vi "camera mjpeg.vi"(11 "CameraDevRef":T1) -> ()   [LabVIEW 2013]
uses:
  <vilib>/Rock Robotics/WPI/Camera/WPI_CameraDevRef.ctl
  <vilib>/Rock Robotics/WPI/Camera/WPI_CameraSettings Operations.ctl
  typedefs/fg_typedef.ctl
  typedefs/Vision/vision enable.ctl
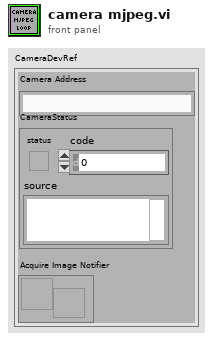
[diagram p1: front panel]
types:
  T1 = typedef "WPI_CameraDevRef.ctl" = cluster{"Camera Address":string, "CameraStatus":errorcluster, "Acquire Image Notifier":refnum<notifier>}
  T2 = typedef "WPI_CameraSettings Operations.ctl" = enum16{"Udate FPS", "Update Compression", "Update Size", "Update White Balance", "Update Brightness", "Update Sharpness", "Update Exposure", "Update Color Level", "Update Exp Priority", "Update Color Enable", "Update JPG", "Update MJPG", "Read and Clear", "Read", "Init"}
  T3 = typedef "vision enable.ctl" = enum16{"Enable", "Disable", "Stop"}
  T4 = typedef "fg_typedef.ctl" = enum16{"Get", "Set"}
  T5 = typedef "WPI_CameraSettings Control.ctl" = cluster{"FPS":i32, "Compression":i32, "Size":i32, "White Balance":i32, "Brightness":i32, "Sharpness":i32, "Exposure":i32, "Color Level":i32, "Exposure Priority":i32, "Color Enable":i32, "JPG Loop":i32, "MJPG Loop":i32}
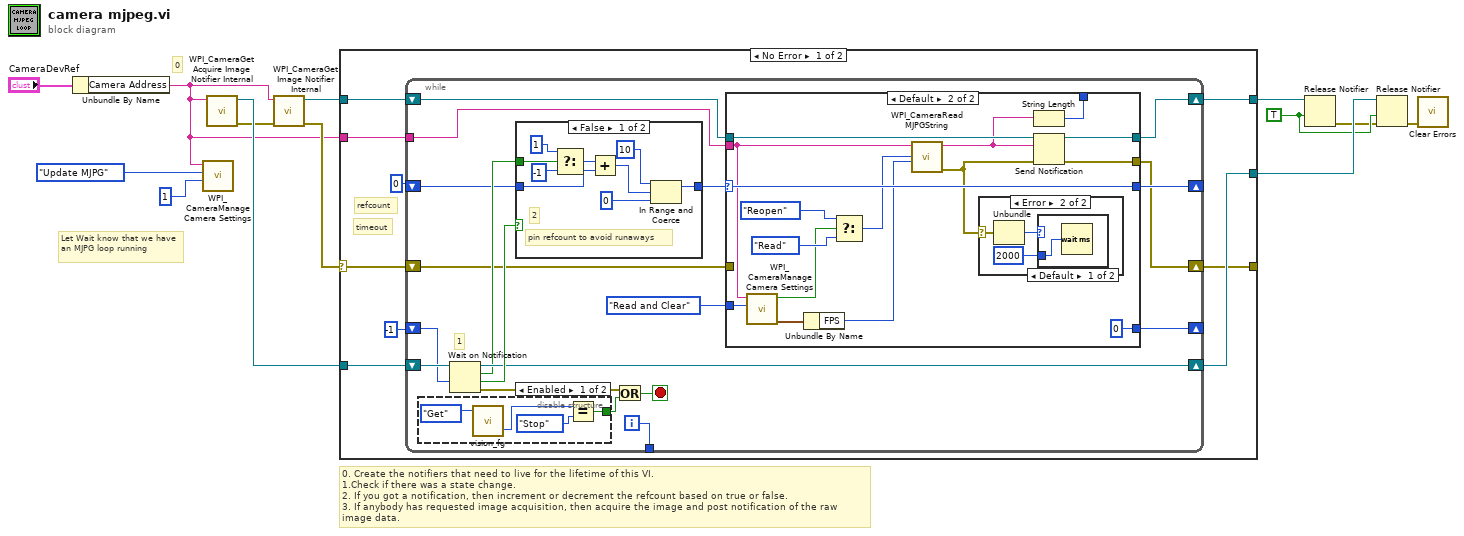
[diagram p0: block diagram]
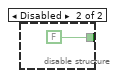
[diagram p2: hidden frame]
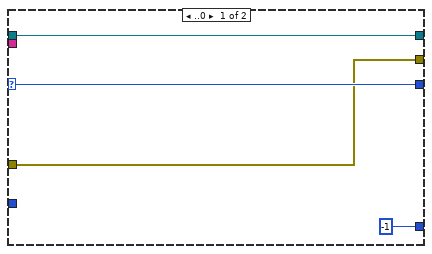
[diagram p3: hidden frame]
diagram:
  w10 = TRUE ("force destroy? (F)")
  # "Let Wait know that we have\nan MJPG loop running"
  # "0"
  # "0. Create the notifiers that need to live for the lifetime of this VI. \n1.Check if there was a state change.\n2. If you got a notification, then increment or decrement the refcount based on true or false.\n3. If anybody has requested image acquisition, then acquire the image and post notification of the raw image data."
  n1 = Unbundle By Name("CameraDevRef") -> ("Camera Address"=w1:string)
  n2 = call <vilib>:"WPI_CameraManage Camera Settings.vi"("Value"=1, "Operation"=WPI_CameraSettings_Operations."Update MJPG", "Camera IP"=w1) -> ()  [unwired: 7 in, 2 out]
  n3 = call <vilib>:"WPI_CameraGet Acquire Image Notifier Internal.vi"("Camera Address"=w1) -> ("error out"=w5:errorcluster, "Acquire Image Notifier"=w6:refnum<notifier>)  [unwired: 1 in, 8 out]
  n4 = call <vilib>:"WPI_CameraGet Image Notifier Internal.vi"("error in (no error)"=w5, "Camera Address"=w1) -> ("error out"=w8:errorcluster, "Image Notifier"=w11:refnum<notifier>)  [unwired: 8 out]
  n5 = case shown="No Error" w8 {
    selector: w8 -> [w15 w83]
    tunnel: w1 -> [w22 _]
    tunnel: w6 -> [w21 w81]
    tunnel: w11 -> [w19 w82]
    tunnel: [w17 w82] -> w13
    tunnel: [w16 w81] -> w12
    tunnel: [w14 w83] -> _
    frame No Error {
      # "timeout"
      # "refcount"
      n6 = while {
        shift-right: [w39] -> w16
        shift-left: w21 -> [w41]
        tunnel: w22 -> [w36]
        shift-right: [w29] -> _
        shift-left: 0 -> [w37]
        shift-right: [w34] -> w17
        shift-left: w19 -> [w35]
        shift-right: [w32] -> _
        shift-left: -1 -> [w33]
        shift-right: [w28] -> w14
        shift-left: w15 -> [w31]
        tunnel: [w26] -> _
        i -> [w26]
        stop <- w25 stop-if-true
        # "1"
        n7 = disable-structure shown="Enabled" {
          disable-tunnel: [w42 FALSE] -> w23
          frame Enabled {
            n8 = call "vision_fg.vi"("Menu"=fg_typedef."Get") -> ("State Out"=w44:T3)  [unwired: 2 in, 1 out]
            n9 = Equal?(x=w44, y=vision_enable."Stop") -> (x = y?=w42:bool)
          }
          frame Disabled {
          }
        }
        n10 = Wait on Notification(notifier=w41, timeout in ms (-1)=w33) -> (notifier out=w39:refnum<notifier>, notification=w38:bool, timed out?=w40:bool, error out=w24:errorcluster)  [unwired: 1 in, 1 out]
        n11 = case shown="False" w40 {
          tunnel: w38 -> [w79 _]
          tunnel: w37 -> [w75 w80]
          tunnel: [w71 w80] -> w30
          frame False {
            # "pin refcount to avoid runaways"
            # "2"
            n12 = Select(t=1, s=w79, f=-1) -> (s? t:f=w76:i32)
            n13 = Add(x=w76, y=w75) -> (x+y=w72:i32)
            n14 = In Range and Coerce(upper limit=10, x=w72, lower limit=0) -> (coerced(x)=w71:i32)  [unwired: 1 out]
          }
          frame True {
          }
        }
        n15 = Or(x=w24, y=w23) -> (x .or. y?=w25:bool)
        n16 = case shown="Default" w30 {
          selector: w30 -> [w49 w63]
          tunnel: w36 -> [_ w51]
          tunnel: w35 -> [w50 w66]
          tunnel: [w50 w65] -> w34
          tunnel: [-1 0] -> w32
          tunnel: w31 -> [w47 _]
          tunnel: [w49 w63] -> w29
          tunnel: [w47 w62] -> w28
          tunnel: [_ w56] -> _
          tunnel: WPI_CameraSettings_Operations."Read and Clear" ("Operation") -> [_ w52]
          frame ..0 {
          }
          frame Default {
            n17 = call <vilib>:"WPI_CameraManage Camera Settings.vi"("Operation"=w52, "Camera IP"=w51) -> ("Values"=w54:T5, "Changed"=w55:bool)  [unwired: 8 in]
            n18 = Unbundle By Name(w54) -> ("FPS"=w53:i32)
            n19 = Select(t=enum16{"Read", "Reopen", "Close"}."Reopen" ("Operation"), s=w55, f=enum16{"Read", "Reopen", "Close"}."Read" ("Operation")) -> (s? t:f=w58:enum16{"Read", "Reopen", "Close"})
            n20 = call <vilib>:"WPI_CameraRead MJPGString.vi"("fps"=w53, "Operation"=w58, "address"=w51) -> ("error out"=w61:errorcluster, "Raw Image Data"=w57:string)  [unwired: 7 in]
            n21 = case shown="Error" w61 {
              selector: w61 -> [_ w69]
              frame No Error {
              }
              frame Error {
                n22 = Unbundle(w69) -> ("code"=w68:i32)  [unwired: 2 out]
                n23 = case shown="Default" w68 {
                  tunnel: u32 2000 ("milliseconds to wait") -> [w70 _]
                  frame Default {
                    n24 = Wait (ms)(milliseconds to wait=w70) -> ()  [unwired: 1 out]
                  }
                  frame 56 {
                  }
                }
              }
            }
            n25 = String Length(string=w57) -> (length=w56:i32)
            n26 = Send Notification(notification=w57, notifier=w66, error in (no error)=w61) -> (notifier out=w65:refnum<notifier>, error out=w62:errorcluster)
          }
        }
      }
    }
    frame Error {
    }
  }
  n27 = Release Notifier(notifier=w13, force destroy? (F)=w10) -> (error out=w4:errorcluster)  [unwired: 1 in, 2 out]
  n28 = Release Notifier(notifier=w12, force destroy? (F)=w10, error in (no error)=w4) -> (error out=w7:errorcluster)  [unwired: 2 out]
  n29 = call <vilib>:"Clear Errors.vi"("error in (no error)"=w7) -> ()  [unwired: 7 out]
